vi "TCPConnectSendRead.vi"(2 "模式（标准）":T1(ring), 4 "数据输入":string, 5 "发送超时(ms)":i32=6000, 6 "读取超时(ms)":i32=6000, 7 "读取的字节":i32=500, 8 "远程端口或服务名称":u16, 9 "地址":string) -> (0 "连接ID输出":refnum<k5>, 1 "错误输出":errorcluster, 3 "数据输出":string)   [LabVIEW 2020]
panel:
  in  "连接超时(ms)":i32=6000
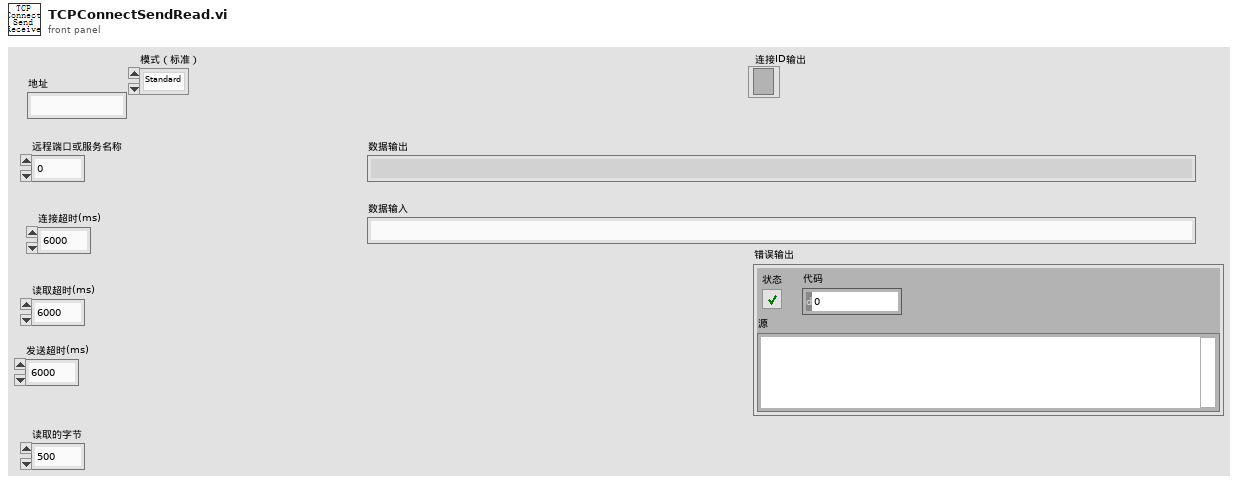
[diagram p1: front panel]
types:
  T1 = enum16{"Standard", "Buffered", "CRLF", "Immediate"}
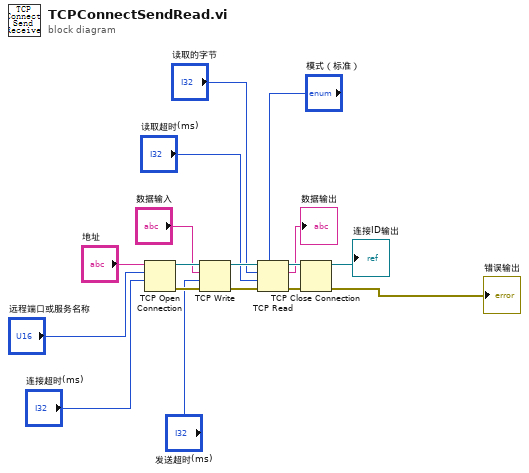
[diagram p0: block diagram]
diagram:
  n1 = TCP Open Connection(address="地址", remote port or service name="远程端口或服务名称", timeout ms (60000)="连接超时(ms)") -> (connection ID=w17:refnum<k5>, error out=w14:errorcluster)  [unwired: 2 in]
  n2 = TCP Write(connection ID=w17, data in="数据输入", error in (no error)=w14, 9:"发送超时(ms)") -> (connection ID out=w16:refnum<k5>, error out=w13:errorcluster)  [unwired: 1 out]
  n3 = TCP Read(connection ID=w16, bytes to read="读取的字节", error in (no error)=w13, 7:"模式（标准）", 9:"读取超时(ms)") -> (connection ID out=w15:refnum<k5>, data out=→"数据输出":string, error out=w12:errorcluster)
  n4 = TCP Close Connection(connection ID=w15, error in (no error)=w12) -> (connection ID out=→"连接ID输出":refnum<k5>, error out=→"错误输出":errorcluster)  [unwired: 1 in]
